vi "FTS CycleCountingWavemeter.vi"(6 "readWrite":enum16{"read", "write"}(ring), 8 "error in":errorcluster, 9 "cycleCounting":bool, 10 "channel index interferogram":u16, 11 "spectrometerIdx":u16) -> (0 "error out":errorcluster, 1 "cycleCounting read":bool, 3 "FTSLib_status":i32)   [LabVIEW 2010, in "OSA.lvclass"]
uses:
  _OSA_class/OSA.lvclass
  FTSLib.dll
panel:
  in  "ignore range violation (false)":bool
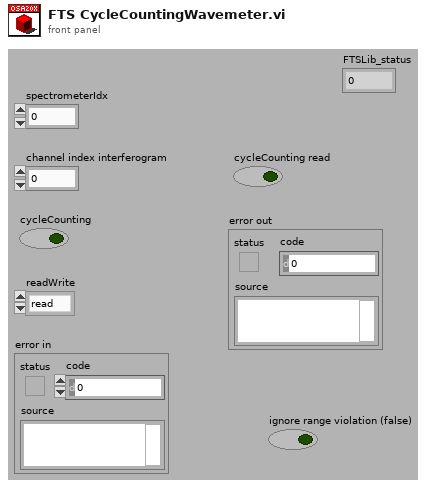
[diagram p1: front panel]
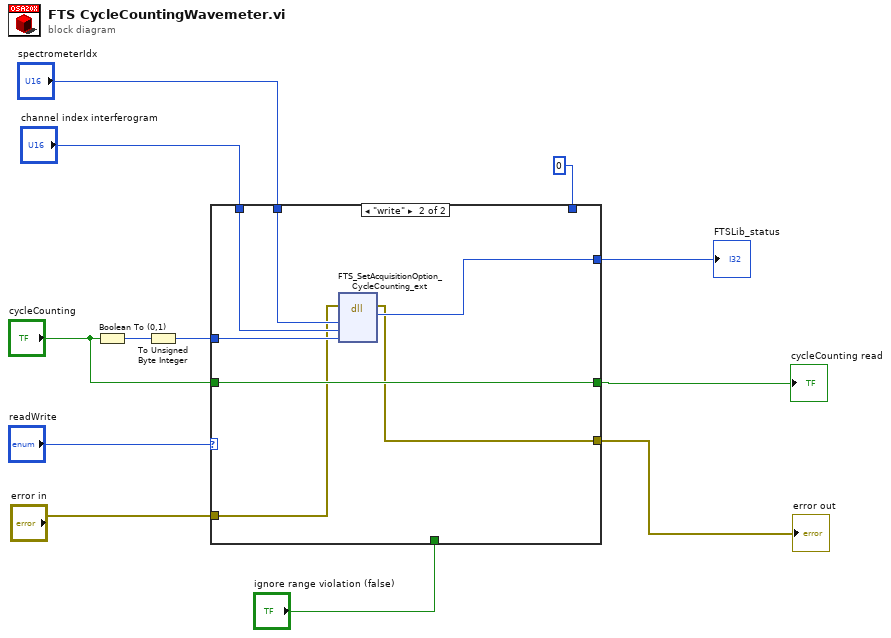
[diagram p0: block diagram]
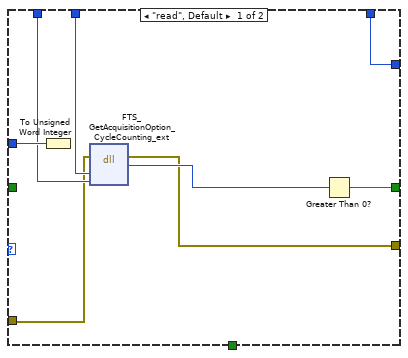
[diagram p2: hidden frame]
diagram:
  n1 = Boolean To (0,1)(Boolean="cycleCounting") -> (0, 1=w7:i16)
  n2 = To Unsigned Byte Integer(number=w7) -> (unsigned 8bit integer=w8:u8)
  n3 = case shown="\"write\"" "readWrite" {
    tunnel: "spectrometerIdx" -> [w20 w27]
    tunnel: w8 -> [w19 w26]
    tunnel: "error in" -> [w15 w22]
    tunnel: "ignore range violation (false)" -> [_ _]
    tunnel: "cycleCounting" -> [_ w25]
    tunnel: [w18 w25] -> w11
    tunnel: [w14 w21] -> w10
    tunnel: "channel index interferogram" -> [w17 w24]
    tunnel: [w13 w23] -> w2
    tunnel: 0 ("return type") -> [w13 _]
    frame "read", Default {
      n4 = To Unsigned Word Integer(number=w19) -> ()  [unwired: 1 out]
      n5 = dll-call lib="FTSLib.dll" fn="FTS_GetAcquisitionOption_CycleCounting_ext"(error in=w15, "spectrIdx"=w20, "channel"=w17) -> (error out=w14:errorcluster, "return type"=w16:i32)  [unwired: 4 in, 1 out]
      n6 = Greater Than 0?(x=w16) -> (x > 0?=w18:bool)
    }
    frame "write" {
      n7 = dll-call lib="FTSLib.dll" fn="FTS_SetAcquisitionOption_CycleCounting_ext"(error in=w22, "spectrIdx"=w27, "channel"=w24, "cycleCounting"=w26) -> (error out=w21:errorcluster, "return type"=w23:i32)  [unwired: 5 in, 1 out]
    }
  }
  "cycleCounting read" <- w11
  "error out" <- w10
  "FTSLib_status" <- w2
